vi "题目5.vi"() -> ()   [LabVIEW 2017]
panel:
  in  "停止":bool
  in  "控制面板":T1 {"档位" scale=0.0..6.0; "油门" scale=0.0..10.0}
  out "显示面板":T2 {"油量" scale=0.0..200.0; "速度" scale=0.0..300.0; "转速" scale=0.0..8000.0}
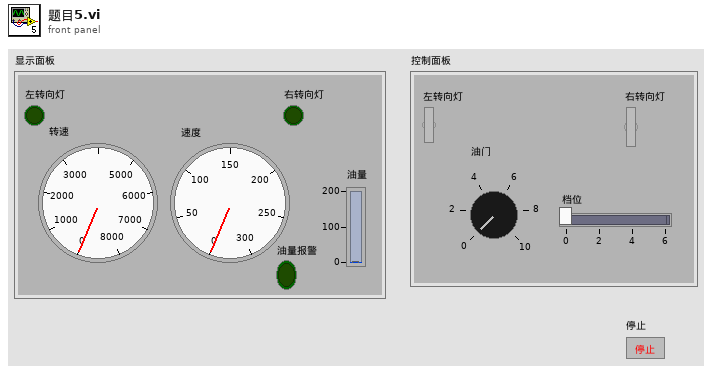
[diagram p1: front panel]
types:
  T1 = cluster{"左转向灯":bool, "右转向灯":bool, "油门":dbl, "档位":dbl}
  T2 = cluster{"左转向灯":bool, "右转向灯":bool, "转速":dbl, "速度 ":dbl, "油量":dbl, "油量报警":bool}
  T3 = cluster{"左转向灯":bool, "右转向灯":bool, dbl, dbl, dbl, bool}
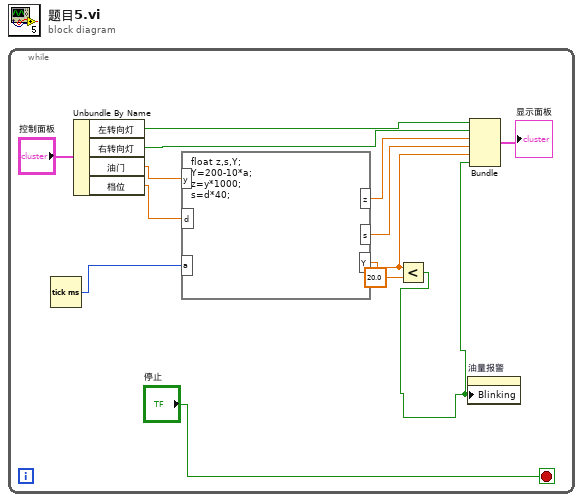
[diagram p0: block diagram]
diagram:
  n1 = while {
    stop <- "停止" stop-if-true
    n2 = Tick Count (ms)() -> (millisecond timer value=w9:u32)
    n3 = Unbundle By Name("控制面板") -> ("左转向灯"=w8:bool, "右转向灯"=w7:bool, "油门"=w11:dbl, "档位"=w10:dbl)
    n4 = formula code="float z,s,Y;\nY=200-10*a;\nz=y*1000;\ns=d*40;"("y"=w11, "d"=w10, "a"=w9) -> ("z"=w2:dbl, "s"=w3:dbl, "Y"=w4:dbl)
    n5 = Less?(x=w4, y=20.0) -> (x < y?=w5:bool)
    n6 = property on="油量报警" class="Bool (严格)"("Blinking"=w5) -> ()  [unwired: 2 in, 2 out]
    n7 = Bundle("左转向灯"=w8, "右转向灯"=w7, w2, w3, w4, w5) -> (→"显示面板":T3)  [unwired: 1 in]
  }
